vi "Zone-to-color_correspondence_lookup_test.vi"() -> ()   [LabVIEW 2018]
panel:
  out "Time per hour, s":dbl
  out "Array 3":u32[](array[numeric])
  out "Array 2":i32[][](array[numeric])
  out "Speed, us per loop":dbl
  out "Array":u32[][](array[colorbox])
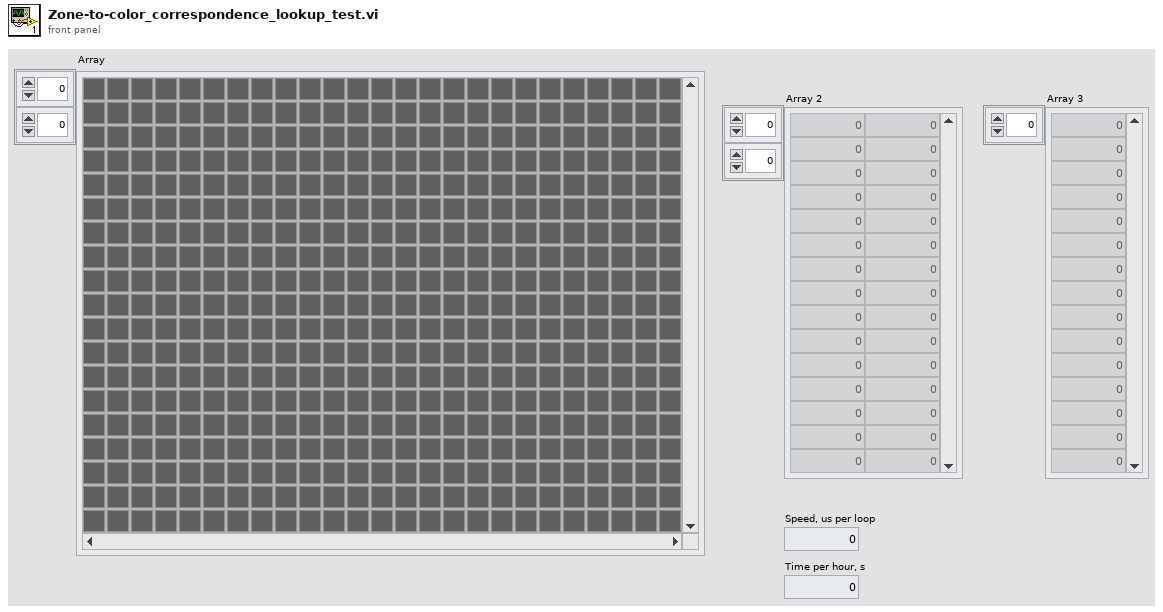
[diagram p1: front panel]
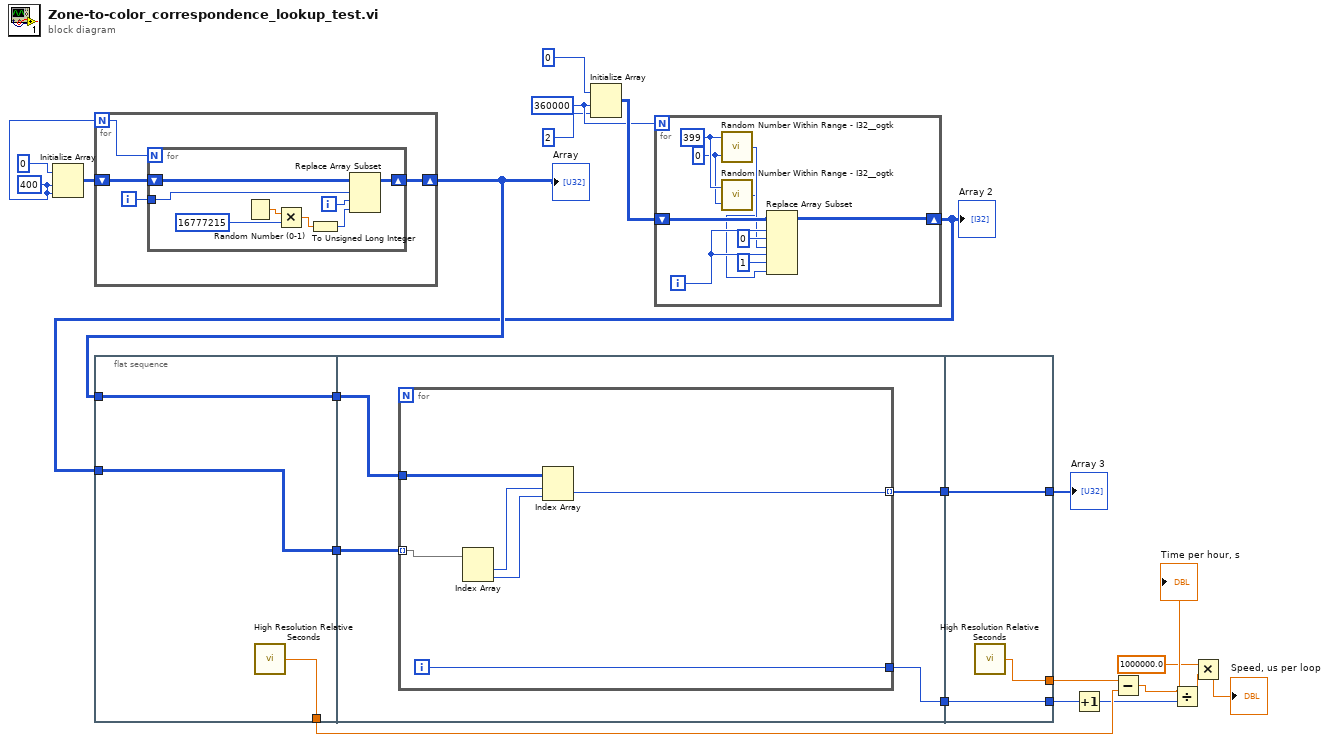
[diagram p0: block diagram]
diagram:
  w9 = 360000 ("dimension size")
  w20 = 400 ("dimension size")
  n1 = Initialize Array(u32 0, w20, w20) -> (w21:u32[][])
  n2 = for {
    N: w20 -> [w23]
    shift-right: [w24] -> w19
    shift-left: w21 -> [w26]
    i -> [w25]
    n3 = for {
      N: w23 -> [_]
      tunnel: w25 -> [w31]
      shift-right: [w28] -> w24
      shift-left: w26 -> [w32]
      i -> [w30]
      n4 = Random Number (0-1)() -> (number: 0 to 1=w34:dbl)
      n5 = Multiply(x=w34, y=u32 16777215) -> (x*y=w33:dbl)
      n6 = To Unsigned Long Integer(number=w33) -> (unsigned 32bit integer=w29:u32)
      n7 = Replace Array Subset(array=w32, new element=w29, index (row)=w31, index (col)=w30) -> (w28:u32[][])
    }
  }
  "Array" <- w19
  n8 = flat-sequence {
    tunnel: w19 -> [w37]
    tunnel: [w37] -> w18
    tunnel: [w36] -> w16
    tunnel: [w35] -> w4
    tunnel: w3 -> [w35]
    tunnel: w18 -> [w41]
    tunnel: [w40] -> w6
    tunnel: w4 -> [w39]
    tunnel: [w38] -> w2
    tunnel: [w50] -> w17
    tunnel: [w49] -> w7
    tunnel: w6 -> [w49]
    tunnel: [w48] -> w1
    tunnel: w2 -> [w48]
    frame #0 {
      n9 = call <vilib>:"High Resolution Relative Seconds.vi"() -> ("relative seconds"=w36:dbl)
    }
    frame #1 {
      n10 = for {
        tunnel: w41 -> [w46]
        tunnel: [w47] -> w40
        tunnel: w39 -> [w45] mode=indexing
        tunnel: [w42] -> w38 mode=indexing
        i -> [w47]
        n11 = Index Array(array=w45) -> (element #1=w44:i32, element #2=w43:i32)  [unwired: 2 in]
        n12 = Index Array(array=w46, index (row)=w44, index (col)=w43) -> (element=w42:u32)
      }
    }
    frame #2 {
      n13 = call <vilib>:"High Resolution Relative Seconds.vi"() -> ("relative seconds"=w50:dbl)
    }
  }
  n14 = Initialize Array(0, w9, 2 ("dimension size")) -> (w10:i32[][])
  n15 = for {
    N: w9 -> [_]
    shift-right: [w58] -> w3
    shift-left: w10 -> [w59]
    i -> [w57]
    w54 = 399 ("High")
    w53 = 0 ("Low")
    n16 = call <userlib>:"Random Number Within Range - I32__ogtk.vi"("High"=w54, "Low"=w53) -> ("Random Number"=w52:i32)  [unwired: 3 in]
    n17 = call <userlib>:"Random Number Within Range - I32__ogtk.vi"("High"=w54, "Low"=w53) -> ("Random Number"=w51:i32)  [unwired: 3 in]
    n18 = Replace Array Subset(array=w59, new element #1=w52, index (row) #1=w57, index (col) #1=0 ("disabled index (col)"), new element #2=w51, index (row) #2=w57, index (col) #2=1 ("disabled index (col)")) -> (w58:i32[][])
  }
  "Array 2" <- w3
  n19 = Increment(x=w7) -> (x+1=w5:i32)
  n20 = Subtract(x=w17, y=w16) -> (x-y=w15:dbl)
  "Time per hour, s" <- w15
  n21 = Divide(x=w15, y=w5) -> (x/y=w14:dbl)
  n22 = Multiply(x=1000000.0, y=w14) -> (x*y=→"Speed, us per loop":dbl)
  "Array 3" <- w1
